vi "_Yt13_SimpleGenericTest.vi"(11 "YTESTER测试数据":T1 caption="不要修改！") -> (3 "YTESTER结论":T2)   [LabVIEW 2017]
doc: "VIClassID=YT_SSTEPFLAG_SIMPLETEST2\nVIDescription=由YYLL开发的通用简易串口测试步骤。。。"
uses:
  YtCommon.lvlibp/yt`Step StepBaseInput.ctl
  Step`s VIs/YYLLIdea/yylltestresult/yylltestresult basis.ctl
  YtCommon.lvlibp/yt`Step StepResult.ctl
  YtCommon.lvlibp/yt`Step TestData.ctl
  YtCommon.lvlibp/yt`Step System Queue.ctl
  Step`s VIs/YYLLGeneric/variable_W.ctl
  YtCommon.lvlibp/yt`Data-Ytester Type Data.ctl
  YtCommon.lvlibp
panel:
  in  "YTESTER开放参数":T5={"YTESTER_BaseInput"={"isTest"=TRUE, "isSkip"=FALSE, "StepName"="简易串口测试", "OnPass"=enum."Next", "OnFail"=enum."Next", "ReTestNumber"=3.0}, "VISA resource"="", "工作模式"=enum."先发后收", "发送字符串"="", "Smart发送预处理"=[], "接收延迟前&发送前清缓存"=TRUE, "接收前延迟ms"=100, "应答检测"="", "应答≥长度检测"=0, "Smart解析预处理"=[], "解析后到变量(自定义建议#开头)"="不到变量", "合格依据"=enum."强制合格", "StringLimit-A"="", "UpperLimit-B"=0.0, "LowLimit-C"=0.0, "unit"="", "明码LOG"=FALSE}
  # "简易通用串口测试步骤"
  # "重入！"
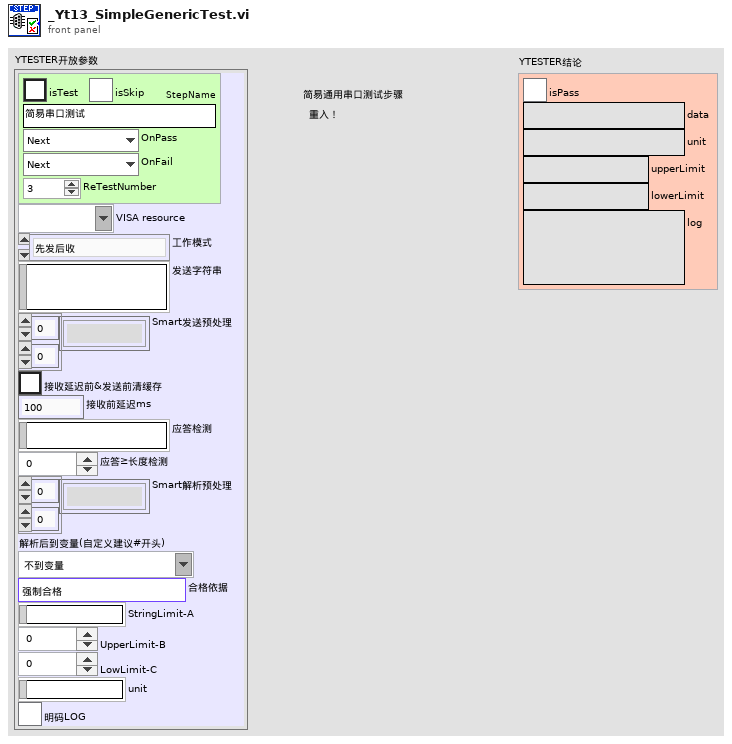
[diagram p1: front panel]
types:
  T1 = typedef "YtCommon.lvlibp/yt`Step TestData.ctl" = cluster{"Socket(From1)":i32, "SN":refnum<notifier>, "StopFlagRef":refnum<notifier>, "YT System Queue":refnum<queue>}
  T2 = typedef "YtCommon.lvlibp/yt`Step StepResult.ctl" = cluster{"isPass":bool, "data":string, "unit":string, "upperLimit":string, "lowerLimit":string, "log":string}
  T3 = typedef "YtCommon.lvlibp/yt`Step StepBaseInput.ctl" = cluster{"isTest":bool, "isSkip":bool, "StepName":string, "OnPass":enum16{"Next", "ToOVER", "Terminate"}, "OnFail":enum16{"Next", "ToOVER", "Terminate"}, "ReTestNumber":dbl}
  T4 = typedef "yylltestresult basis.ctl" = enum16{"强制合格", "强制不合格", "随机合格", "X=A", "X=\"真\"", "X=\"假\"", "X≠A", "X包含A", "X不包含A", "A包含X", "A包含非空X", "A不包含X", "X等于A正则匹配内容", "X包含A正则匹配内容", "X不包含A正则匹配内容", "X=B", "X≠B", "X＞B", "X≥B", "X＜B", "X≤B", "B≥X≥C", "B≥X＞C", "B＞X≥C", "B＞X＞C", "X≥B | C≥X", "X＞B | C≥X", "X≥B | C＞X", "X＞B | C＞X"}
  T5 = cluster{"YTESTER_BaseInput":T3, "VISA resource":refnum<visa-resource-name>, "工作模式":enum16{"先发后收", "仅发送", "仅接收"}, "发送字符串":string, "Smart发送预处理":string[][], "接收延迟前&发送前清缓存":bool, "接收前延迟ms":u32, "应答检测":string, "应答≥长度检测":i32, "Smart解析预处理":string[][], "解析后到变量(自定义建议#开头)":string, "合格依据":T4, "StringLimit-A":string, "UpperLimit-B":dbl, "LowLimit-C":dbl, "unit":string, "明码LOG":bool}
  T6 = typedef "variable_W.ctl" = cluster{"YT_TYPE":T7, "TypeData":string[], "Tips":string}
  T7 = typedef "YtCommon.lvlibp/yt`Data-Ytester Type Data.ctl" = enum16{"NULL", "NUM", "BOOL", "TXT", "ENUM", "TIME", "PATH", "VISA", "COMBO", "ColorBox", "RadioBtn", "Array_NUM", "Array_BOOL", "Array_TXT", "Array_ENUM", "Array_PATH", "Array_COMBO"}
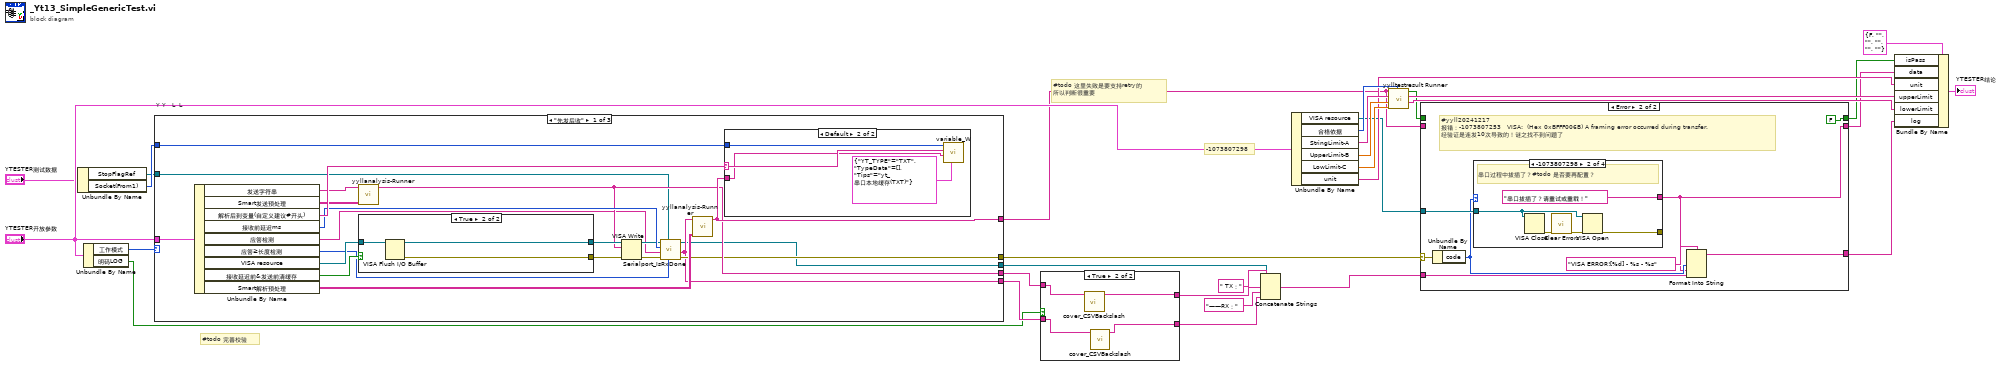
[diagram p0: block diagram]
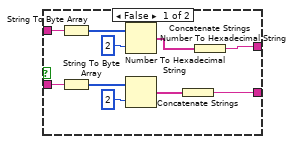
[diagram p2: hidden frame]
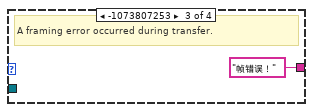
[diagram p5: hidden frame]
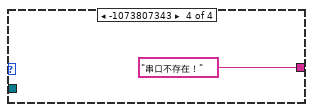
[diagram p6: hidden frame]
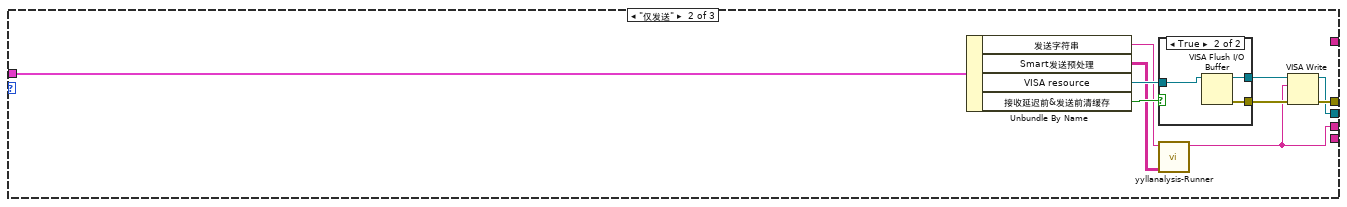
[diagram p9: hidden frame]
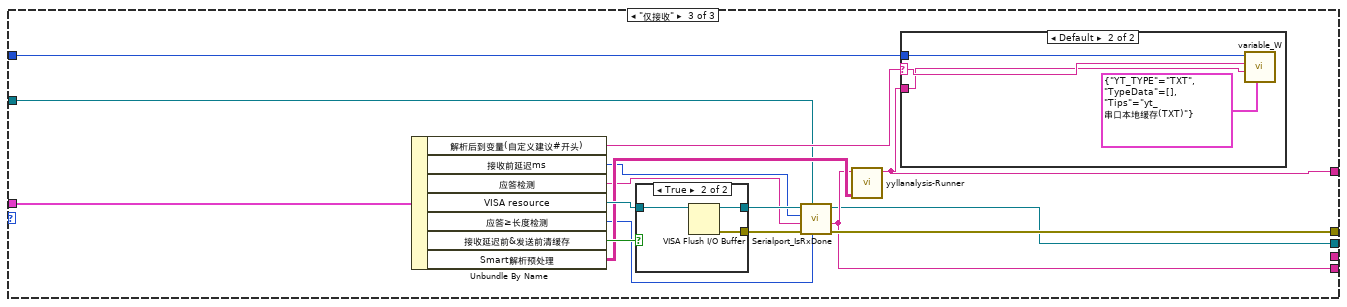
[diagram p11: hidden frame]
diagram:
  # "Y Y   L  L"
  # "-1073807298"
  # "#todo 完善校验"
  # "#todo 这里失败是要支持retry的\n所以判断很重要"
  n1 = Unbundle By Name("YTESTER测试数据") -> ("StopFlagRef"=w12:refnum<notifier>, "Socket(From1)"=w27:i32)
  n2 = Unbundle By Name("YTESTER开放参数") -> ("工作模式"=w28:enum16{"先发后收", "仅发送", "仅接收"}, "明码LOG"=w1:bool)
  n3 = case shown="\"先发后收\"" w28 {
    tunnel: "YTESTER开放参数" -> [w51 w69 w89]
    tunnel: [w36 w68 w79] -> w10
    tunnel: w27 -> [w48 _ w87]
    tunnel: [w40 w61 _] -> w25
    tunnel: [w35 _ w76] -> w24
    tunnel: [w42 _ w83] -> w6
    tunnel: w12 -> [w38 _ w82]
    tunnel: [w34 w60 w75] -> w2
    frame "先发后收" {
      n4 = Unbundle By Name(w51) -> ("发送字符串"=w45:string, "Smart发送预处理"=w44:string[][], "解析后到变量(自定义建议#开头)"=w47:string, "接收前延迟ms"=w41:u32, "应答检测"=w32:string, "应答≥长度检测"=w31:i32, "VISA resource"=w50:refnum<visa-resource-name>, "接收延迟前&发送前清缓存"=w46:bool, "Smart解析预处理"=w43:string[][])
      n5 = call "yyllanalysis-Runner.vi"("inputs"=w44, "String in"=w45) -> ("String out"=w40:string)  [unwired: 8 in, 1 out]
      n6 = case shown="True" w46 {
        tunnel: w50 -> [w52 w55]
        tunnel: [w52 w54] -> w49
        tunnel: [_ w53] -> w39
        frame False {
        }
        frame True {
          n7 = VISA Flush I/O Buffer(VISA resource name=w55) -> (VISA resource name out=w54:refnum<visa-resource-name>, error out=w53:errorcluster)  [unwired: 2 in]
        }
      }
      n8 = VISA Write(VISA resource name=w49, write buffer=w40, error in (no error)=w39) -> (VISA resource name out=w37:refnum<visa-resource-name>, error out=w33:errorcluster)  [unwired: 1 out]
      n9 = call "Serialport_IsRxDone.vi"("应答长度检测"=w31, "StopFlagRef"=w38, "error in (no error)"=w33, "应答检测"=w32, "接收前延迟ms"=w41, "VISA"=w37) -> ("error out"=w36:errorcluster, "Rx"=w35:string, "VISA out"=w34:refnum<visa-resource-name>)  [unwired: 2 in, 1 out]
      n10 = call "yyllanalysis-Runner.vi"("inputs"=w43, "String in"=w35) -> ("String out"=w42:string)  [unwired: 8 in, 1 out]
      n11 = case shown="Default" w47 {
        selector: w47 -> [_ w58]
        tunnel: w48 -> [_ w59]
        tunnel: w42 -> [_ w57]
        frame "不到变量" {
        }
        frame Default {
          n12 = call "variable_W.vi"("附加的Information"=T6 {"YT_TYPE"=enum."TXT", "TypeData"=[], "Tips"="yt_串口本地缓存(TXT)"}, "待写入池的输入控件"=w57, "待写入池变量名称"=w58, "函数池名称 in"=w59) -> ()  [unwired: 5 in, 3 out]
        }
      }
    }
    frame "仅发送" {
      n13 = Unbundle By Name(w69) -> ("发送字符串"=w63:string, "Smart发送预处理"=w62:string[][], "VISA resource"=w66:refnum<visa-resource-name>, "接收延迟前&发送前清缓存"=w67:bool)
      n14 = case shown="True" w67 {
        tunnel: w66 -> [w70 w73]
        tunnel: [w70 w72] -> w65
        tunnel: [_ w71] -> w64
        frame False {
        }
        frame True {
          n15 = VISA Flush I/O Buffer(VISA resource name=w73) -> (VISA resource name out=w72:refnum<visa-resource-name>, error out=w71:errorcluster)  [unwired: 2 in]
        }
      }
      n16 = call "yyllanalysis-Runner.vi"("inputs"=w62, "String in"=w63) -> ("String out"=w61:string)  [unwired: 8 in, 1 out]
      n17 = VISA Write(VISA resource name=w65, write buffer=w61, error in (no error)=w64) -> (VISA resource name out=w60:refnum<visa-resource-name>, error out=w68:errorcluster)  [unwired: 1 out]
    }
    frame "仅接收" {
      n18 = Unbundle By Name(w89) -> ("解析后到变量(自定义建议#开头)"=w88:string, "接收前延迟ms"=w78:u32, "应答检测"=w77:string, "VISA resource"=w85:refnum<visa-resource-name>, "应答≥长度检测"=w74:i32, "接收延迟前&发送前清缓存"=w86:bool, "Smart解析预处理"=w84:string[][])
      n19 = case shown="True" w86 {
        tunnel: w85 -> [w90 w93]
        tunnel: [w90 w92] -> w81
        tunnel: [_ w91] -> w80
        frame False {
        }
        frame True {
          n20 = VISA Flush I/O Buffer(VISA resource name=w93) -> (VISA resource name out=w92:refnum<visa-resource-name>, error out=w91:errorcluster)  [unwired: 2 in]
        }
      }
      n21 = call "Serialport_IsRxDone.vi"("应答长度检测"=w74, "StopFlagRef"=w82, "error in (no error)"=w80, "应答检测"=w77, "接收前延迟ms"=w78, "VISA"=w81) -> ("error out"=w79:errorcluster, "Rx"=w76:string, "VISA out"=w75:refnum<visa-resource-name>)  [unwired: 2 in, 1 out]
      n22 = call "yyllanalysis-Runner.vi"("inputs"=w84, "String in"=w76) -> ("String out"=w83:string)  [unwired: 8 in, 1 out]
      n23 = case shown="Default" w88 {
        selector: w88 -> [_ w96]
        tunnel: w87 -> [_ w97]
        tunnel: w83 -> [_ w95]
        frame "不到变量" {
        }
        frame Default {
          n24 = call "variable_W.vi"("附加的Information"=T6 {"YT_TYPE"=enum."TXT", "TypeData"=[], "Tips"="yt_串口本地缓存(TXT)"}, "待写入池的输入控件"=w95, "待写入池变量名称"=w96, "函数池名称 in"=w97) -> ()  [unwired: 5 in, 3 out]
        }
      }
    }
  }
  n25 = case shown="True" w1 {
    tunnel: [w99 w108] -> w26
    tunnel: w25 -> [w104 w109]
    tunnel: w24 -> [w101 w111]
    tunnel: [w98 w110] -> w21
    frame False {
      n26 = String To Byte Array(string=w104) -> (unsigned byte array=w106:u8[])
      n27 = String To Byte Array(string=w101) -> (unsigned byte array=w102:u8[])
      n28 = Number To Hexadecimal String(1:i16 2 ("width (-)"), 2:w106) -> (0:w107:string[])
      n29 = Number To Hexadecimal String(1:i16 2 ("width (-)"), 2:w102) -> (0:w100:string[])
      n30 = Concatenate Strings(w100) -> (w98:string)
      n31 = Concatenate Strings(w107) -> (w99:string)
    }
    frame True {
      n32 = call "cover_CSVBackslash.vi"("String in"=w109) -> ("String out"=w108:string)  [unwired: 10 in]
      n33 = call "cover_CSVBackslash.vi"("String in"=w111) -> ("String out"=w110:string)  [unwired: 10 in]
    }
  }
  n34 = Concatenate Strings(w2, " TX：", w26, "——RX：", w21) -> (w3:string)
  n35 = Unbundle By Name("YTESTER开放参数") -> ("VISA resource"=w7:refnum<visa-resource-name>, "合格依据"=w19:T4, "StringLimit-A"=w18:string, "UpperLimit-B"=w17:dbl, "LowLimit-C"=w16:dbl, "unit"=w15:string)
  n36 = call "yylltestresult Runner.vi"("合格依据"=w19, "LowLimit-C"=w16, "UpperLimit-B"=w17, "StringLimit-A"=w18, "DataIn-X"=w6) -> ("lowerLimit"=w13:string, "upperLimit"=w14:string, "isPass"=w8:bool)  [unwired: 4 in]
  n37 = case shown="Error" w10 {
    selector: w10 -> [_ w121]
    tunnel: [w114 FALSE ("isPass")] -> w9
    tunnel: w8 -> [w114 _]
    tunnel: w7 -> [_ w120]
    tunnel: [w113 w116] -> w5
    tunnel: w6 -> [w113 _]
    tunnel: [w112 w117] -> w4
    tunnel: w3 -> [w112 w115]
    frame No Error {
    }
    frame Error {
      # "#yyll20241217  \n报错：-1073807253   VISA:  (Hex 0xBFFF006B) A framing error occurred during transfer.\n经验证是连发10次导致的！谜之找不到问题了"
      n38 = Unbundle By Name(w121) -> ("code"=w119:i32)
      n39 = case shown="-1073807298" w119 {
        tunnel: w120 -> [_ w126 _ _]
        tunnel: [_ w124 _ _] -> _
        tunnel: [_ "串口拔插了？请重试或重载！" "帧错误！" "串口不存在！"] -> w116
        frame 0, Default {
        }
        frame -1073807298 {
          # "串口过程中拔插了？#todo 是否要再配置？"
          n40 = VISA Close(VISA resource name=w126) -> (error out=w127:errorcluster)  [unwired: 1 in]
          n41 = call <vilib>:"Clear Errors.vi"("error in (no error)"=w127) -> ("error out"=w125:errorcluster)  [unwired: 5 in, 1 out]
          n42 = VISA Open(error in (no error)=w125, VISA resource name=w126) -> (error out=w124:errorcluster)  [unwired: 3 in, 1 out]
        }
        frame -1073807253 {
          # "A framing error occurred during transfer."
        }
        frame -1073807343 {
        }
      }
      n43 = Format Into String(format string="VISA ERROR![%d] - %s - %s", w119, w116, w115) -> (resulting string=w117:string)  [unwired: 2 in, 1 out]
    }
  }
  n44 = Bundle By Name(cluster=T2 {"isPass"=FALSE, "data"="", "unit"="", "upperLimit"="", "lowerLimit"="", "log"=""} ("Result"), "isPass"=w9, "data"=w5, "unit"=w15, "upperLimit"=w14, "lowerLimit"=w13, "log"=w4) -> (→"YTESTER结论":T2)
